vi "LoadAndRun_byName_VEPS.vi"(4 "error in (no error)":errorcluster, 5 "data-control name":string, 6 "run?":bool, 7 "path":path) -> (0 "error out":errorcluster, 2 "data-control refnum out":refnum<vi>, 3 "vi refnum out":refnum<vi>)   [LabVIEW 2011]
doc: "Opens a refnum to the specified VI and, optionally, runs it. It will also return a reference to the first control whose name is the specified string."
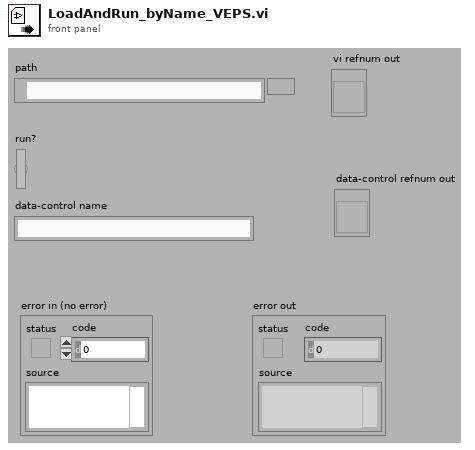
[diagram p1: front panel]
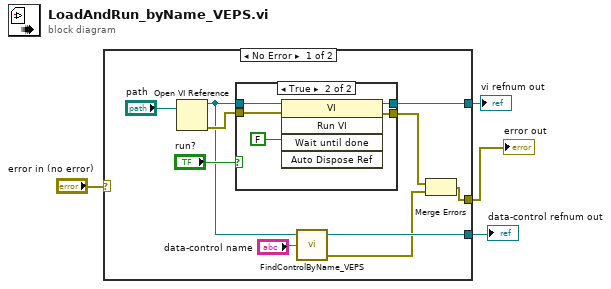
[diagram p0: block diagram]
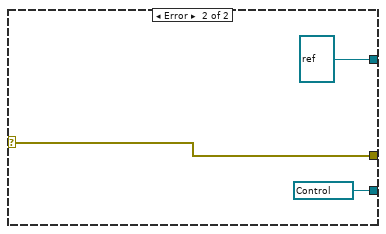
[diagram p3: hidden frame]
diagram:
  n1 = case shown="No Error" "error in (no error)" {
    selector: "error in (no error)" -> [_ w23]
    tunnel: [w12 refnum<vi> refnum] -> w3
    tunnel: [w7 w23] -> w2
    tunnel: [w8 refnum<vi> refnum ("control refnum")] -> w1
    frame No Error {
      n2 = Open VI Reference(vi path="path") -> (vi reference=w10:refnum<vi>, error out=w11:errorcluster)  [unwired: 5 in]
      n3 = case shown="True" "run?" {
        tunnel: w10 -> [w16 w21]
        tunnel: [w16 w19] -> w12
        tunnel: w11 -> [w15 w18]
        tunnel: [w15 w17] -> w6
        frame False {
        }
        frame True {
          n4 = invoke class="VI" method="Run VI"(reference=w21, error in=w18, "Wait until done"=FALSE) -> (reference out=w19:refnum<vi>, error out=w17:errorcluster)  [unwired: 2 in, 3 out]
        }
      }
      n5 = call "FindControlByName_VEPS.vi"("control name"="data-control name", "vi refnum"=w10) -> ("error out"=w5:errorcluster, "control refnum"=w8:refnum<vi>)  [unwired: 2 in]
      n6 = Merge Errors(w6, w5) -> (w7:errorcluster)
    }
    frame Error {
    }
  }
  "vi refnum out" <- w3
  "error out" <- w2
  "data-control refnum out" <- w1
